vi "VI Refs Loader.vi"(7 "Config File Path":path) -> (4 "Setup Name":string, 8 "VI Path/Ref":T1(array[cluster]), 15 "VIs Loaded?":bool)   [LabVIEW 2016]
panel:
  out "Paths to Load":string[](array[string])
  out "File Lines":string[](array[string])
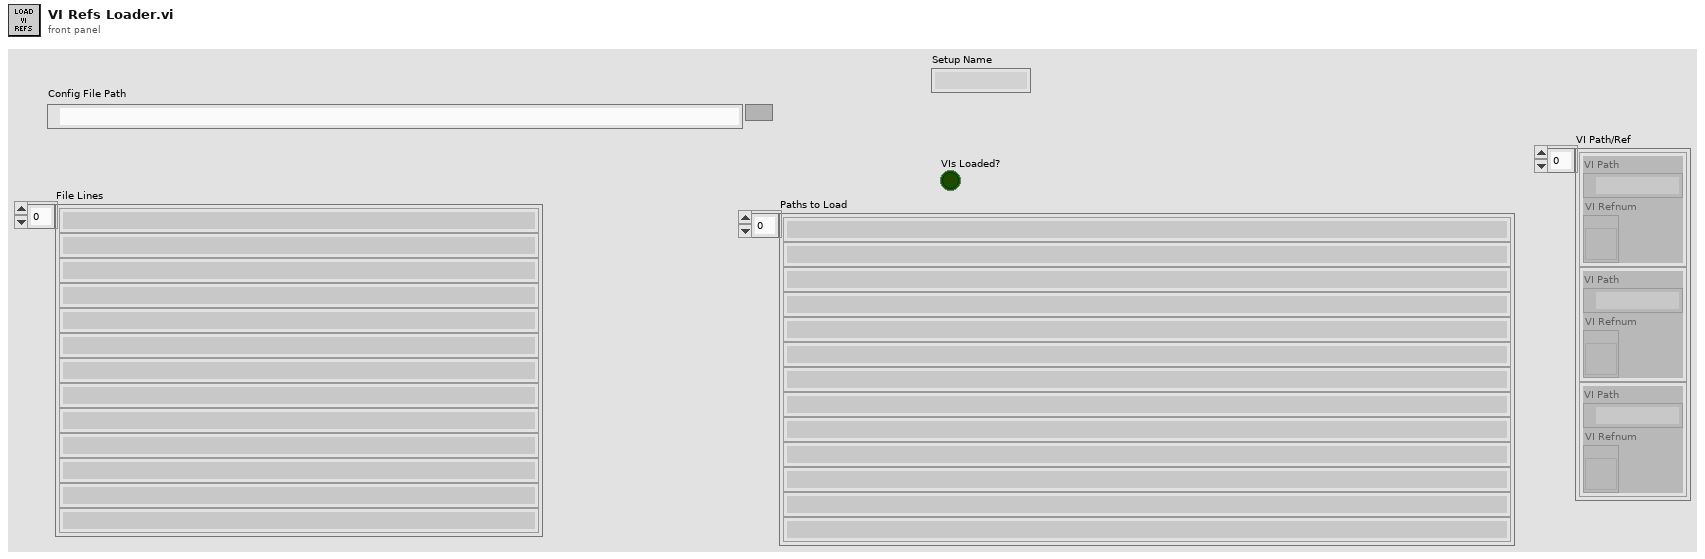
[diagram p1: front panel]
types:
  T1 = cluster{"VI Path":path, "VI Refnum":refnum<vi>}[]
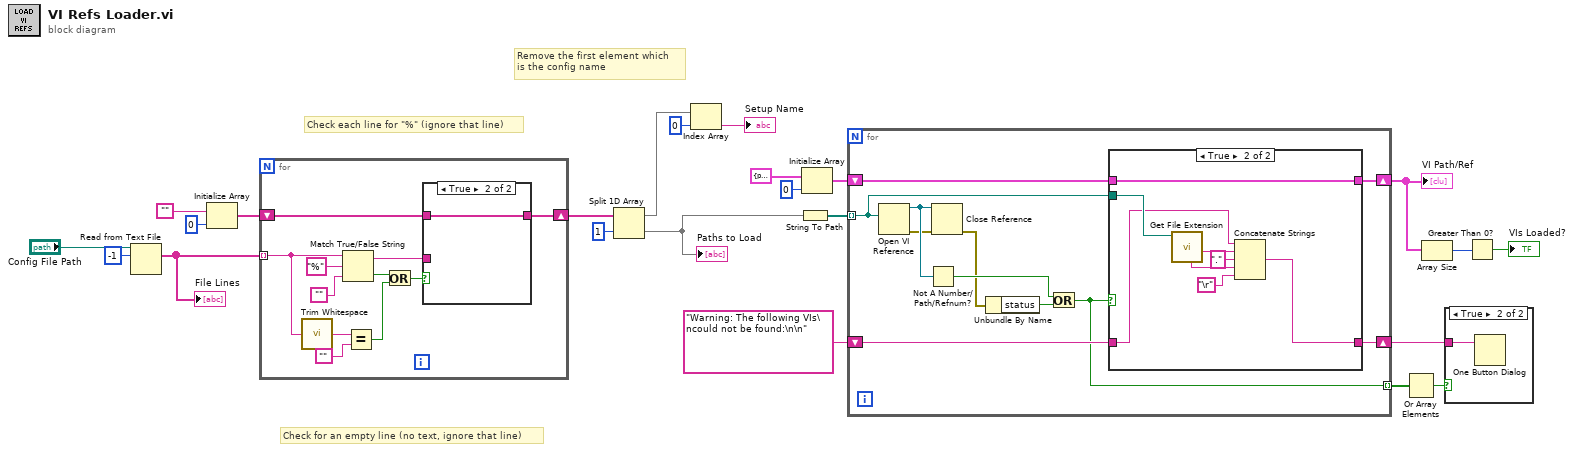
[diagram p0: block diagram]
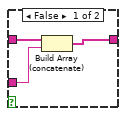
[diagram p2: hidden frame]
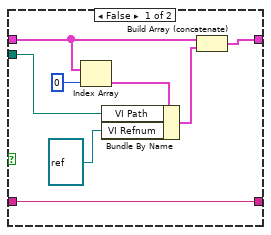
[diagram p4: hidden frame]
diagram:
  # "Remove the first element which\nis the config name"
  # "Check for an empty line (no text, ignore that line)"
  # "Check each line for \"%\" (ignore that line)"
  n1 = Read from Text File(file (use dialog)="Config File Path", count=-1) -> (text=w11:string[])  [unwired: 2 in, 3 out]
  "File Lines" <- w11
  n2 = Initialize Array("", 0 ("dimension size")) -> (w8:string[])
  n3 = for {
    tunnel: w11 -> [w29] mode=indexing
    shift-right: [w31] -> w6
    shift-left: w8 -> [w32]
    n4 = call <vilib>:"Trim Whitespace.vi"("string"=w29) -> ("trimmed string"=w28:string)  [unwired: 1 in]
    n5 = Match True/False String(2:"", 3:"%" ("true string"), 4:w29) -> (0:w26:bool, 1:w33:string)
    n6 = Equal?(x=w28, y="") -> (x = y?=w25:bool)
    n7 = Or(x=w26, y=w25) -> (x .or. y?=w24:bool)
    n8 = case shown="True" w24 {
      tunnel: w33 -> [w35 _]
      tunnel: w32 -> [w37 w38]
      tunnel: [w36 w38] -> w31
      frame False {
        n9 = Build Array (concatenate)(w37, w35) -> (w36:string[])
      }
      frame True {
      }
    }
  }
  n10 = Split 1D Array(array=w6, index=1) -> (first subarray=w3:string[], second subarray=w4:string[])
  "Paths to Load" <- w4
  n11 = Index Array(array=w3, index=0) -> (element=→"Setup Name":string)
  n12 = String To Path(string=w4) -> (path=w22:path[])
  n13 = Initialize Array(cluster{"VI Path":path, "VI Refnum":refnum<vi>} {"VI Path"=path "", "VI Refnum"=refnum}, 0 ("dimension size")) -> (w16:T1)
  n14 = for {
    tunnel: w22 -> [w43] mode=indexing
    shift-right: [w42] -> w20
    shift-left: w16 -> [w47]
    shift-right: [w40] -> w14
    shift-left: "Warning: The following VIs\ncould not be found:\n\n" -> [w41]
    tunnel: [w39] -> w13 mode=indexing
    n15 = Open VI Reference(vi path=w43) -> (vi reference=w46:refnum<vi>, error out=w45:errorcluster)  [unwired: 5 in]
    n16 = Not A Number/Path/Refnum?(number/path/refnum=w46) -> (NaN/Path/Refnum?=w49:bool)
    n17 = Close Reference(reference=w46, error in (no error)=w45) -> (error out=w44:errorcluster)
    n18 = Unbundle By Name(w44) -> ("status"=w48:bool)
    n19 = Or(x=w49, y=w48) -> (x .or. y?=w39:bool)
    n20 = case shown="True" w39 {
      tunnel: w47 -> [w56 w65]
      tunnel: [w57 w65] -> w42
      tunnel: w43 -> [w51 w61]
      tunnel: w41 -> [w50 w59]
      tunnel: [w50 w58] -> w40
      frame False {
        n21 = Index Array(array=w56, index=0) -> (element=w54:cluster{"VI Path":path, "VI Refnum":refnum<vi>})
        n22 = Bundle By Name(cluster=w54, "VI Path"=w51, "VI Refnum"=refnum<vi> refnum) -> (w52:cluster{"VI Path":path, "VI Refnum":refnum<vi>})
        n23 = Build Array (concatenate)(w56, w52) -> (w57:T1)
      }
      frame True {
        n24 = call <vilib>:"Get File Extension.vi"("file"=w61) -> ("filename without extension"=w62:string, "unmodified file extension"=w63:string)  [unwired: 6 in, 3 out]
        n25 = Concatenate Strings(w59, w62, "." ("string"), w63, "\r") -> (w58:string)
      }
    }
  }
  "VI Path/Ref" <- w20
  n26 = Or Array Elements(Boolean array=w13) -> (logical OR=w12:bool)
  n27 = Array Size(array=w20) -> (size(s)=w19:i32)
  n28 = case shown="True" w12 {
    tunnel: w14 -> [_ w66]
    frame False {
    }
    frame True {
      n29 = One Button Dialog(message=w66) -> ()  [unwired: 1 in, 1 out]
    }
  }
  n30 = Greater Than 0?(x=w19) -> (x > 0?=→"VIs Loaded?":bool)
